vi "Configure Channel (RTD Delta).vi"(0 "VISA resource name":refnum<visa-resource-name>, 1 "Reference Channel (0001)":string="0001", 5 "Channel (0001)":string="0001", 7 "Enable Channel (True)":bool=TRUE, 9 "Type and Span":T1={"RTD Type (0 : Pt100)"=0, "Enable Span (False)"=FALSE, "Lower Span (-200.0)"=-200.0, "Upper Span (850.0)"=850.0, "Bias (0)"=0.0} {"Bias (0)" format="%_6g"; "Upper Span (850.0)" min=-99999.0 max=99999.0 step=0.1 format="%.2f"; "Lower Span (-200.0)" min=-99999.0 max=99999.0 step=0.1 format="%.2f"; "RTD Type (0 : Pt100)" items=["Pt100", "Pt100-H", "JPt100", "JPt100-H", "Cu10GE", "Cu10LN", "Cu10WEED", "Cu10BAILEY", "Cu10a392", "Cu10a393", "Cu25", "Cu53", "Cu100", "J263B", "Ni100SAMA", "Ni100DIN", "Ni120", "Pt25", "Pt50", "Pt200WEED", "Cu10G", "Cu50G", "Cu100G", "Pt46G", "Pt100G"]}, 11 "error in (no error)":errorcluster) -> (4 "VISA resource name out":refnum<visa-resource-name>, 6 "Channel":string, 15 "error out":errorcluster)   [LabVIEW 2020, in "Yokogawa GX Series.lvlib"]
doc: "Sets the input range as Resistance Temperature Detector (RTD).\n\nCommand: SRangeAI"
uses:
  <instrlib>/Yokogawa GX Series/Yokogawa GX Series.lvlib
  <instrlib>/Yokogawa GX Series/Private/RTD Range.vi
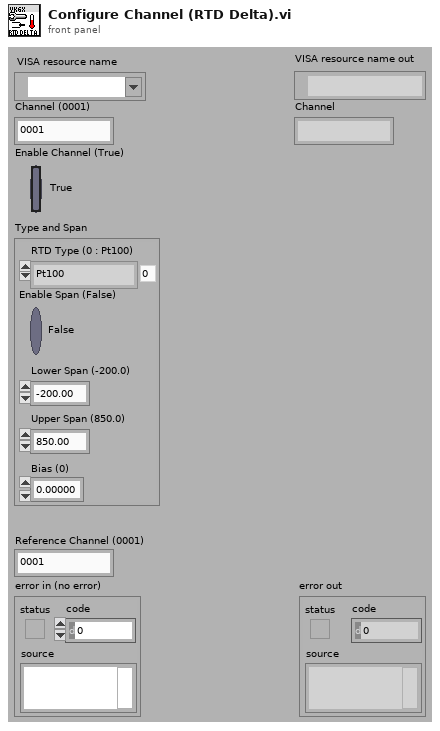
[diagram p1: front panel]
types:
  T1 = cluster{"RTD Type (0 : Pt100)":i32, "Enable Span (False)":bool, "Lower Span (-200.0)":dbl, "Upper Span (850.0)":dbl, "Bias (0)":dbl}
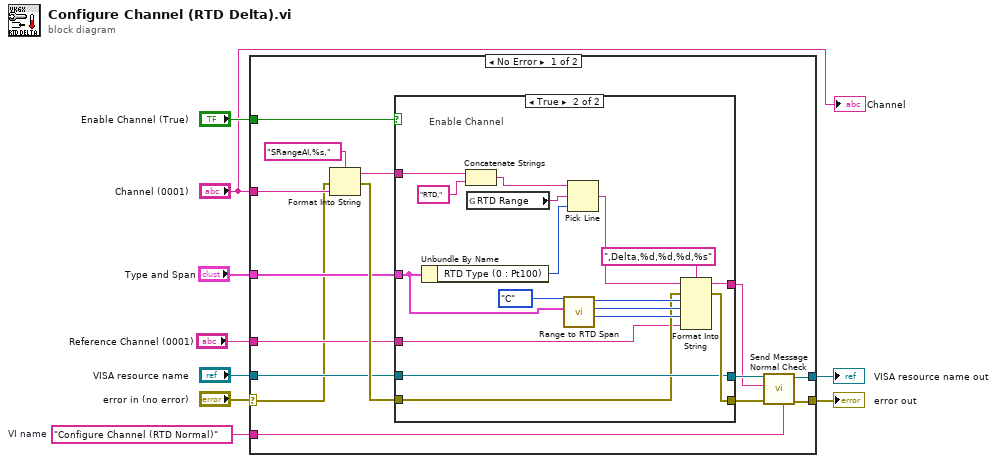
[diagram p0: block diagram]
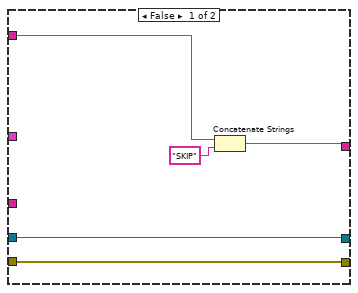
[diagram p2: hidden frame]
diagram:
  w4 = "Configure Channel (RTD Normal)"  # VI name
  n1 = case shown="No Error" "error in (no error)" {
    selector: "error in (no error)" -> [w10 w47]
    tunnel: "Enable Channel (True)" -> [w21 _]
    tunnel: "VISA resource name" -> [w20 w48]
    tunnel: "Type and Span" -> [w19 _]
    tunnel: [w15 w48] -> w6
    tunnel: [w14 w47] -> w5
    tunnel: w4 -> [w13 _]
    tunnel: "Reference Channel (0001)" -> [w12 _]
    tunnel: "Channel (0001)" -> [w11 _]
    frame No Error {
      n2 = Format Into String(format string="SRangeAI,%s,", error in=w10, w11) -> (resulting string=w22:string, error out=w23:errorcluster)  [unwired: 1 in]
      n3 = case shown="True" w21 {
        tunnel: w23 -> [w28 w33]
        tunnel: w22 -> [w29 w45]
        tunnel: [w28 w44] -> w17
        tunnel: w20 -> [w27 w34]
        tunnel: [w27 w34] -> w18
        tunnel: w19 -> [_ w41]
        tunnel: [w25 w38] -> w16
        tunnel: w12 -> [_ w32]
        frame False {
          n4 = Concatenate Strings(w29, "SKIP") -> (w25:string)
        }
        frame True {
          # "Enable Channel"
          n5 = Unbundle By Name(w41) -> ("RTD Type (0 : Pt100)"=w40:i32)
          n6 = Concatenate Strings(w45, "RTD,") -> (w43:string)
          n7 = global read "RTD Range.vi" "RTD Range"() -> (w30:string)
          n8 = call <instrlib>:"Range to RTD Span.vi"("Type and Span"=w41, "Temp. unit (0: C)"=enum16{"C", "F"}."C") -> ("Bias"=w35:i32, "Upper span"=w36:i32, "Lower Span"=w37:i32)  [unwired: 7 in]
          n9 = Pick Line(string ("")=w43, multi-line string=w30, line index=w40) -> (output string=w39:string)
          n10 = Format Into String(format string=",Delta,%d,%d,%d,%s", initial string=w39, error in=w33, w37, w36, w35, w32) -> (resulting string=w38:string, error out=w44:errorcluster)
        }
      }
      n11 = call <instrlib>:"Send Message Normal Check.vi"("Source (\"\")"=w13, "error in (no error)"=w17, "Send Message (\"\")"=w16, "VISA resource name"=w18) -> ("error out"=w14:errorcluster, "VISA resource name out"=w15:refnum<visa-resource-name>)  [unwired: 2 in, 4 out]
    }
    frame Error {
    }
  }
  "error out" <- w5
  "VISA resource name out" <- w6
  "Channel" <- "Channel (0001)"
